vi "Builder-Get Project Info.vi"(0 "Project ref":refnum<vi>, 11 "error in (no error)":errorcluster) -> (4 "Project Path":path, 8 "ProjectItem":refnum<vi>, 15 "error out":errorcluster)   [LabVIEW 2020]
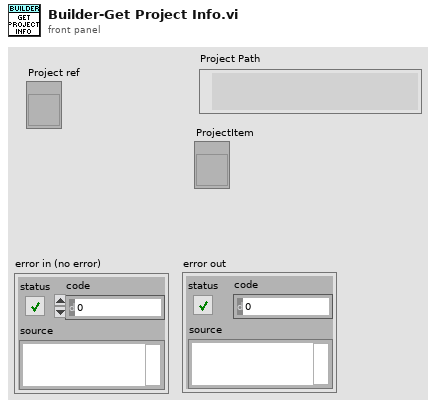
[diagram p1: front panel]
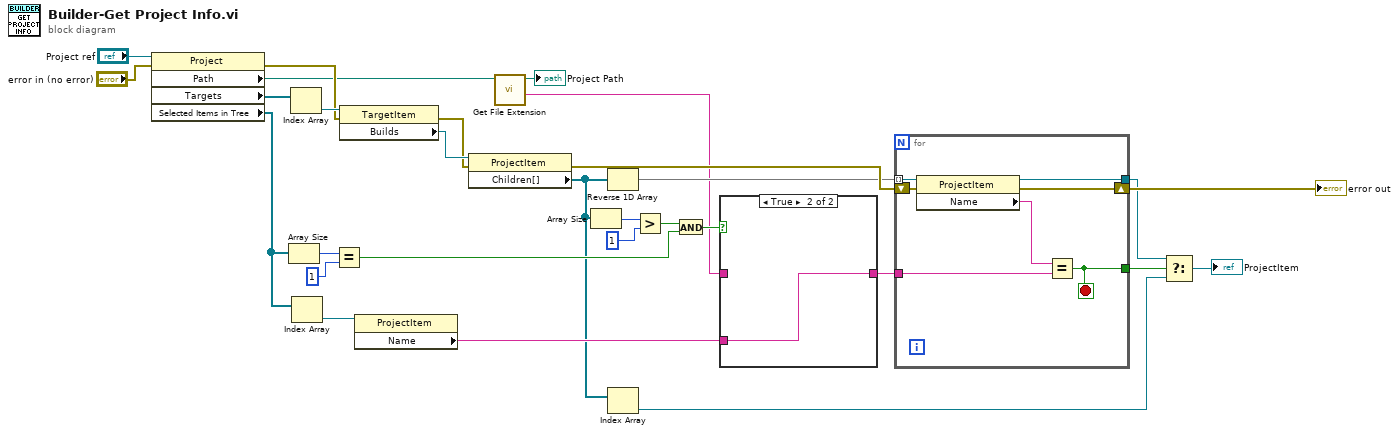
[diagram p0: block diagram]
diagram:
  n1 = property class="Project"(reference="Project ref", error in="error in (no error)") -> (error out=w26:errorcluster, "Path"=w7:path, "Targets"=w29:refnum<vi>[], "Selected Items in Tree"=w12:refnum<vi>[])  [unwired: 1 out]
  n2 = Array Size(array=w12) -> (size(s)=w18:i32)
  n3 = Index Array(array=w29) -> (element=w28:refnum<vi>)  [unwired: 1 in]
  n4 = Index Array(array=w12) -> (element=w11:refnum<vi>)  [unwired: 1 in]
  n5 = Equal?(x=w18, y=1) -> (x = y?=w13:bool)
  n6 = property class="TargetItem"(reference=w28, error in=w26) -> (error out=w24:errorcluster, "Builds"=w25:refnum<vi>)  [unwired: 1 out]
  n7 = property class="ProjectItem"(reference=w11) -> ("Name"=w9:string)  [unwired: 1 in, 2 out]
  n8 = property class="ProjectItem"(reference=w25, error in=w24) -> (error out=w27:errorcluster, "Children[]"=w5:refnum<vi>[])  [unwired: 1 out]
  n9 = call <vilib>:"Get File Extension.vi"("file"=w7) -> ("filename without extension"=w6:string, "dup file"=→"Project Path":path)  [unwired: 6 in, 3 out]
  n10 = Array Size(array=w5) -> (size(s)=w16:i32)
  n11 = Reverse 1D Array(array=w5) -> (reversed array=w22:refnum<vi>[])
  n12 = Index Array(array=w5) -> (element=w2:refnum<vi>)  [unwired: 1 in]
  n13 = Greater?(x=w16, y=1) -> (0:w14:bool)
  n14 = And(x=w14, y=w13) -> (x .and. y?=w10:bool)
  n15 = case shown="True" w10 {
    tunnel: w9 -> [_ w31]
    tunnel: [w30 w31] -> w8
    tunnel: w6 -> [w30 _]
    frame False {
    }
    frame True {
    }
  }
  n16 = for {
    tunnel: w22 -> [w38] mode=indexing
    tunnel: [w36] -> w3
    shift-right: [w34] -> w21
    shift-left: w27 -> [w37]
    tunnel: w8 -> [w33]
    tunnel: [w32] -> w4
    stop <- w32 stop-if-true
    n17 = property class="ProjectItem"(reference=w38, error in=w37) -> (reference out=w36:refnum<vi>, error out=w34:errorcluster, "Name"=w35:string)
    n18 = Equal?(x=w35, y=w33) -> (x = y?=w32:bool)
  }
  "error out" <- w21
  n19 = Select(t=w3, s=w4, f=w2) -> (s? t:f=→"ProjectItem":refnum<vi>)
